vi "Init.vi"(10 "Ini path":path) -> (3 "RESTLoaderIni out":refnum<class "RESTLoaderIni.lvclass">)   [LabVIEW 2019, in "ByteREST.lvlib" / "RESTLoaderIni.lvclass"]
uses:
  RESTLoaderIni.lvclass
  RESTLoaderIni.lvclass/RESTLoaderIni.ctl
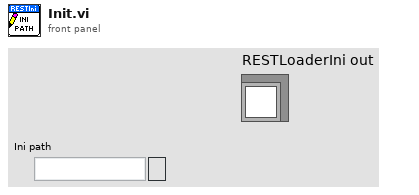
[diagram p1: front panel]
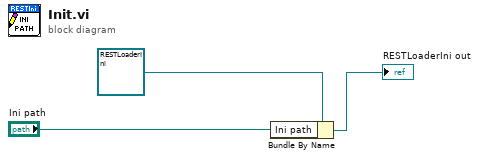
[diagram p0: block diagram]
diagram:
  n1 = Bundle By Name(cluster=refnum<class "RESTLoaderIni.lvclass"> refnum ("RESTLoaderIni in"), "Ini path"="Ini path") -> (→"RESTLoaderIni out":refnum<class "RESTLoaderIni.lvclass">)
